vi "Electrical Measurements - Main.vi"() -> ()   [LabVIEW 2013]
doc: "Use this template to build a standard state machine design pattern. Each state executes code and determines which state to transition to. Contrast this design pattern with the User Interface Event Handler pattern, in which code executes in response to user actions. Contrast this design pattern also with the Queued Message Handler pattern, in which each message handling code can queue zero or more new messages."
uses:
  Controls/StateMachineStates 1.ctl
  Libraries/California Instruments iX Series/California Instruments iX Series.lvlib
  <instrlib>/California Instruments iX Series/Public/Data/Read Multiple Current Measurements.vi
panel:
  out "Waveform Graph":sgl[][](graph)
  out "Current Measurements 2":sgl[](array[numeric])
  out "Current Measurements":sgl[](array[numeric])
  out "multi-line string":string=":MEAS:CURR:AC?\n:MEAS:CURR:CRES?\n:MEAS:CURR:HARM:THD?\n:MEAS:POW:AC:REAL?\n:MEAS:POW:AC:APP?\n:MEAS:POW:AC:REAC?\n:MEAS:POW:AC:PFAC?\n:MEAS:POW:AC:TOT?\n:MEAS:VOLT:AC?\n:MEAS:VOLT:HARM:THD?"
  out "Waveforms":string[](array[string])
  out "Array":dbl[](array[numeric])
  in  "keep reading data/ stop and turn off":bool
  in  "Tab Control":T1(tab)
  in  "Enable Current Protection (Enabled)":bool
  in  "Current Level (0 A)":dbl=2.0
  in  "Current Protection Delay (0.1 Sec)":dbl=0.1
  in  "Voltage Mode (0: Fixed)":i32(ring) items=["Fixed", "Step", "Pulse", "List"]
  in  "Voltage Auto Level Control (0: On)":u16(ring) items=["On", "Off", "Regulation"]
  in  "Voltage Source (0:Internal)":u16(ring) items=["Internal", "External"]
  in  "Voltage Level (0V)":dbl=120.0
  in  "Transient Voltage Level (0V)":dbl
  in  "Voltage Protection Range (150V)":u16(ring)=150 items=["150"=150, "300"=300]
  in  "Voltage Limit (0.0 V)":dbl format="%.2g"
  in  "Phase (0°)":dbl
  in  "Triggered Phase (0°)":dbl
  in  "Phase Mode (0: Fixed)":i32(ring) items=["Fixed", "Step", "Pulse", "List"]
  in  "Frequency (60 Hz)":dbl=60.0
  in  "Triggered Frequency (60 Hz)":dbl=60.0
  in  "Frequency Mode (0: Fixed)":i32(ring) items=["Fixed", "Step", "Pulse", "List", "Sense", "External"]
  in  "Serial Configuration":cluster{"Baud Rate":u32, "Flow Control":u16}={"Baud Rate"=460800, "Flow Control"=0} {"Flow Control" items=["None", "XON/XOFF", "RTS/CTS", "XON/XOFF & RTS/CTS", "DTR/DSR", "XON/XOFF & DTR/DSR"]; "Baud Rate" items=["9600"=9600, "19200"=19200, "38400"=38400, "57600"=57600, "115200"=115200, "230400"=230400, "460800"=460800]}
  in  "VISA resource name":refnum<visa-resource-name>
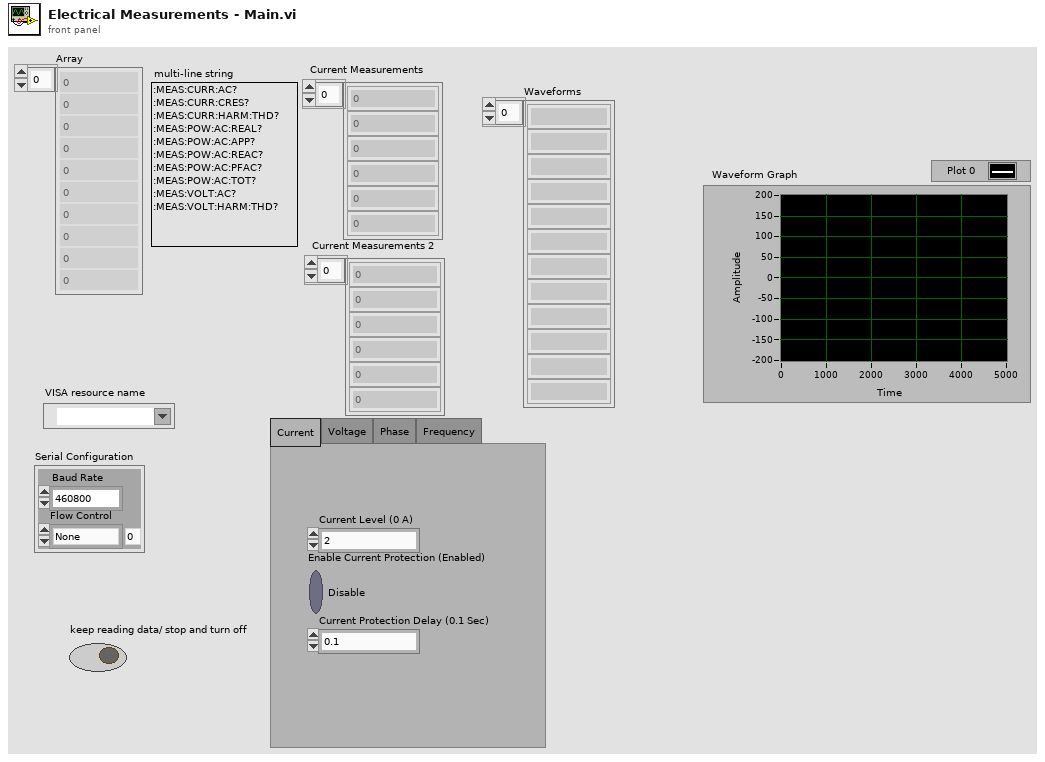
[diagram p1: front panel]
types:
  T1 = enum32{"Current", "Voltage", "Phase", "Frequency"}
  T2 = typedef "StateMachineStates 1.ctl" = enum16{"Idle", "Initialize", "turn supply on", "read electrical data", "read arb wave list", "read waveform data", "turn off light", "Stop"}
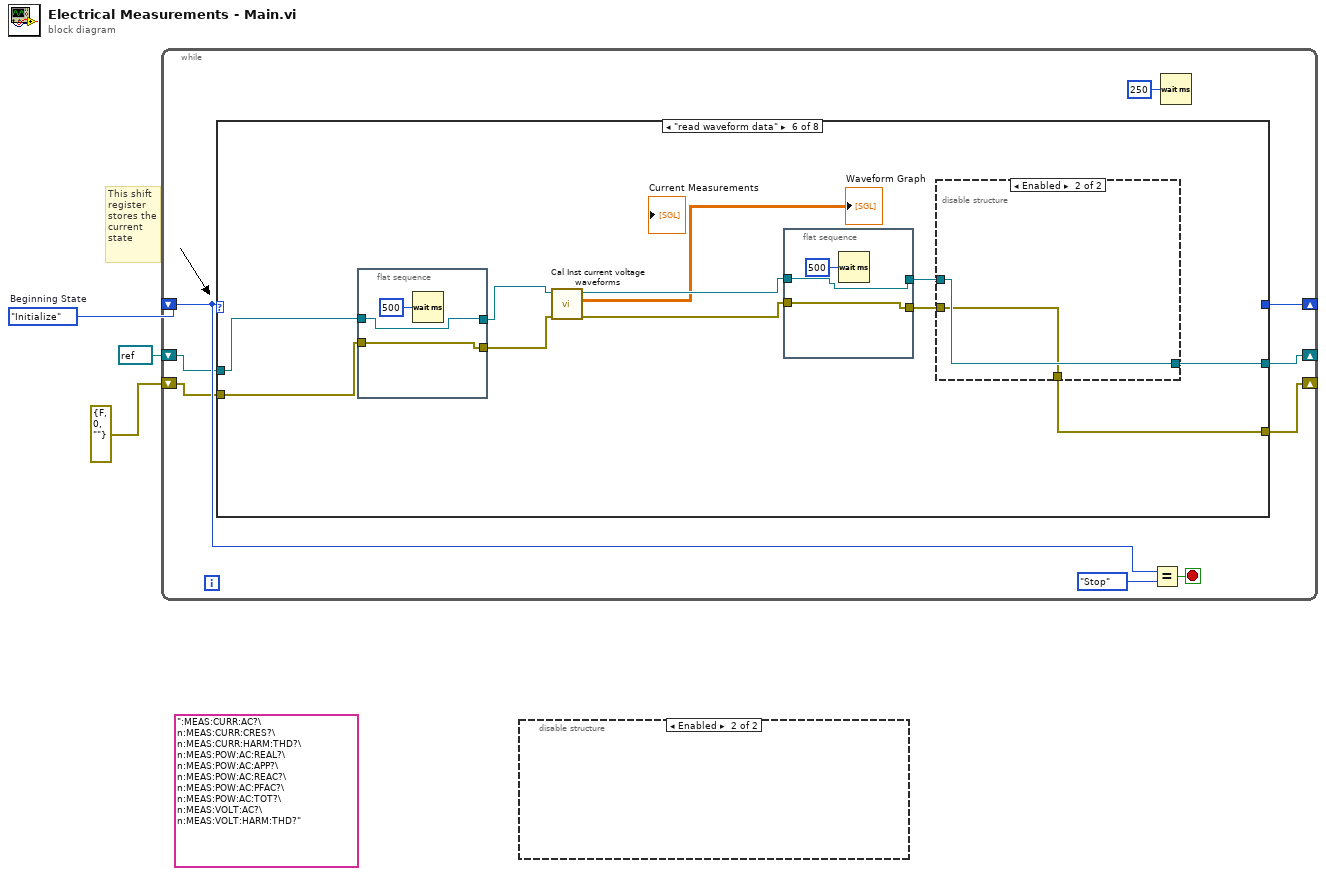
[diagram p0: block diagram]
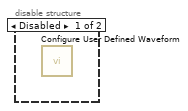
[diagram p2: hidden frame]
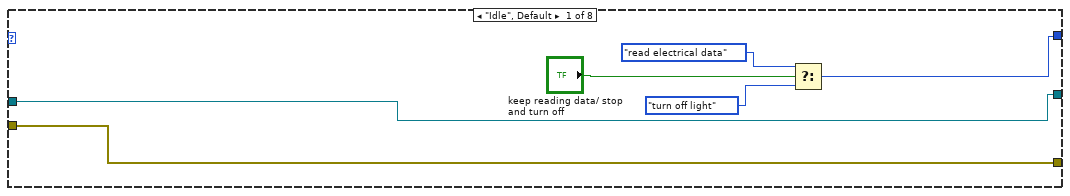
[diagram p3: hidden frame]
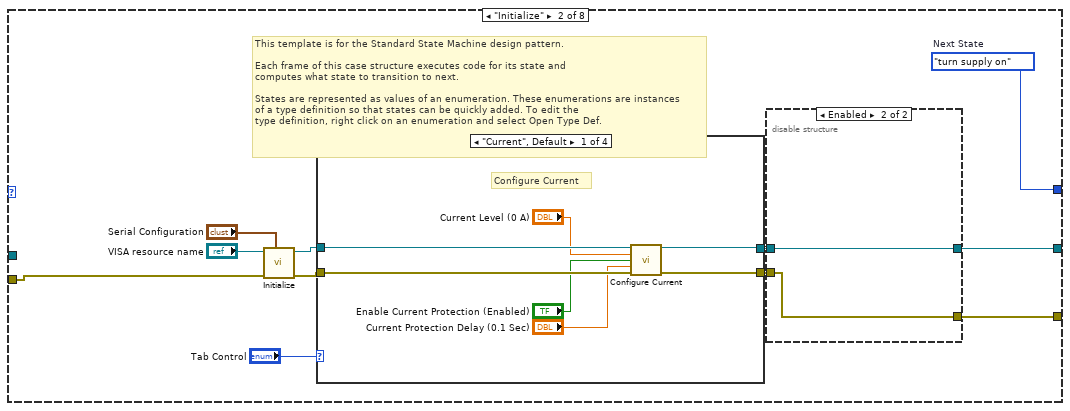
[diagram p4: hidden frame]
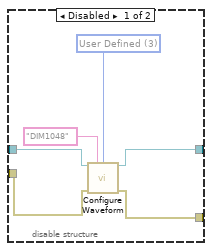
[diagram p5: hidden frame]
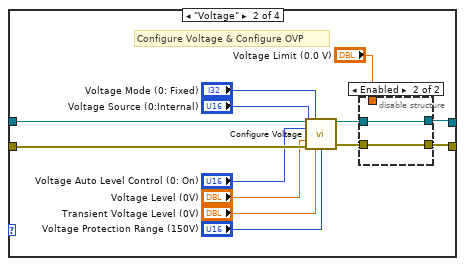
[diagram p6: hidden frame]
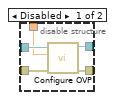
[diagram p7: hidden frame]
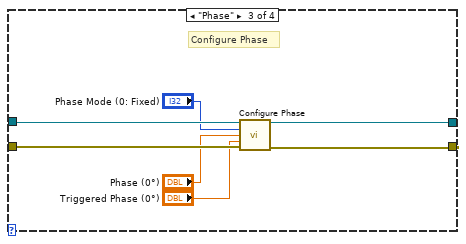
[diagram p8: hidden frame]
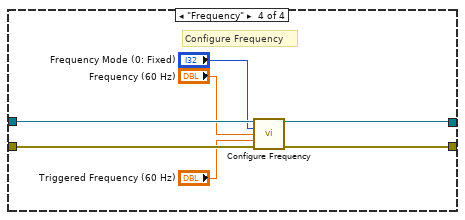
[diagram p9: hidden frame]
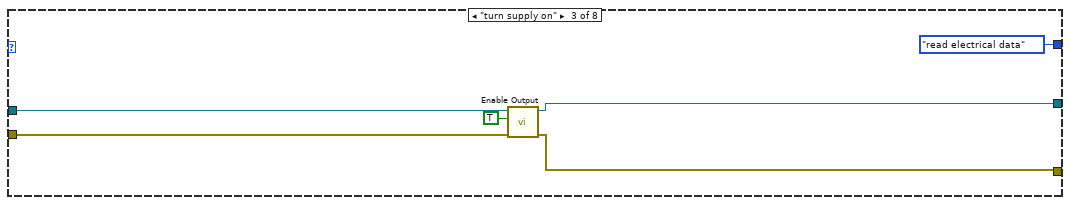
[diagram p10: hidden frame]
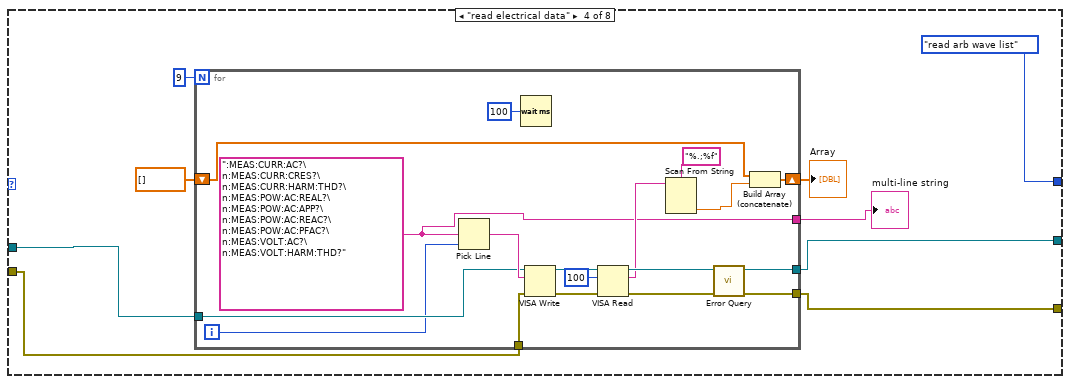
[diagram p11: hidden frame]
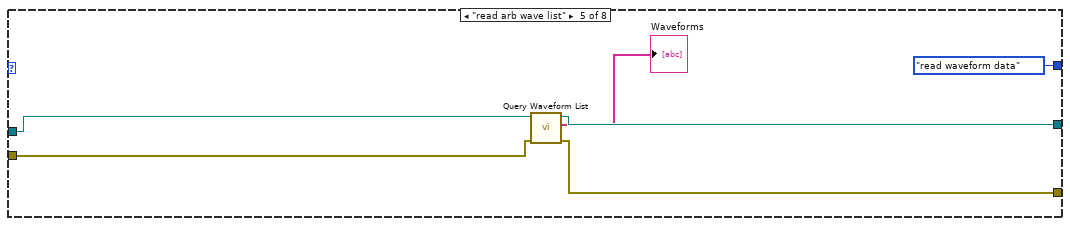
[diagram p12: hidden frame]
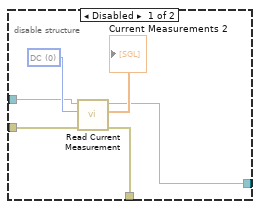
[diagram p13: hidden frame]
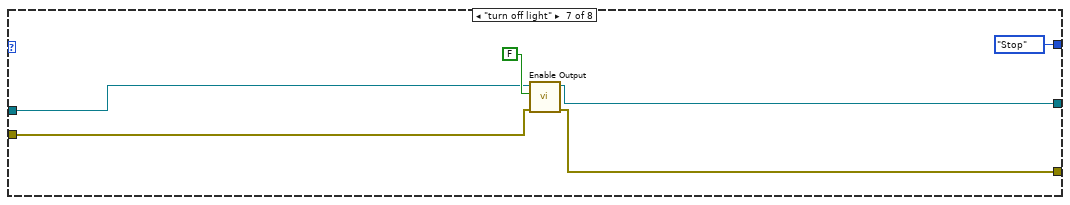
[diagram p14: hidden frame]
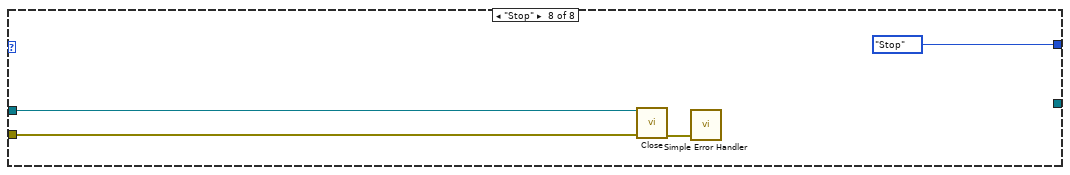
[diagram p15: hidden frame]
diagram:
  (unwired) ":MEAS:CURR:AC?\n:MEAS:CURR:CRES?\n:MEAS:CURR:HARM:THD?\n:MEAS:POW:AC:REAL?\n:MEAS:POW:AC:APP?\n:MEAS:POW:AC:REAC?\n:MEAS:POW:AC:PFAC?\n:MEAS:POW:AC:TOT?\n:MEAS:VOLT:AC?\n:MEAS:VOLT:HARM:THD?" ("multi-line string")
  w3 = StateMachineStates_1."Initialize"  # Beginning State
  # "This shift\nregister\nstores the\ncurrent\nstate"
  n1 = while {
    shift-right: [w9] -> _
    shift-left: w3 -> [w10]
    shift-right: [w5] -> _
    shift-left: refnum<visa-resource-name> refnum ("VISA resource name out") -> [w7]
    shift-right: [w4] -> _
    shift-left: errorcluster {"status"=FALSE, "code"=0, "source"=""} ("error out") -> [w6]
    stop <- w12 stop-if-true
    n2 = case shown="\"read waveform data\"" w10 {
      tunnel: [w15 w29 StateMachineStates_1."read electrical data" ("Next State") StateMachineStates_1."read arb wave list" ("Next State") StateMachineStates_1."read waveform data" ("Next State") _ StateMachineStates_1."Stop" ("Next State") StateMachineStates_1."Stop" ("Next State")] -> w9
      tunnel: w7 -> [w13 _ w84 w92 w117 w124 w145 w150]
      tunnel: w6 -> [w14 w23 w83 w91 w114 w123 w144 w149]
      tunnel: [w13 w20 w80 w89 w116 w126 w147 _] -> w5
      tunnel: [w14 w21 w79 w90 w115 w125 w146 _] -> w4
      frame "Idle", Default {
        n3 = Select(t=StateMachineStates_1."read electrical data" ("Next State"), s="keep reading data/ stop and turn off", f=StateMachineStates_1."turn off light" ("Next State")) -> (s? t:f=w15:T2)
      }
      frame "Initialize" {
        w29 = StateMachineStates_1."turn supply on"  # Next State
        # "This template is for the Standard State Machine design pattern.\n\nEach frame of this case structure executes code for its state and\ncomputes what state to transition to next.\n\nStates are represented as values of an enumeration. These enumerations are instances\nof a type definition so that states can be quickly added. To edit the \ntype definition, right click on an enumeration and select Open Type Def."
        n4 = call "Initialize.vi"("Serial Configuration"="Serial Configuration", "error in (no error)"=w23, "VISA resource name"="VISA resource name") -> ("error out"=w24:errorcluster, "VISA resource name out"=w25:refnum<visa-resource-name>)  [unwired: 7 in]
        n5 = case shown="\"Current\", Default" "Tab Control" {
          tunnel: w25 -> [w44 w57 w71 w78]
          tunnel: w24 -> [w43 w56 w70 w77]
          tunnel: [w39 w46 w66 w73] -> w19
          tunnel: [w38 w45 w65 w72] -> w22
          frame "Current", Default {
            # "Configure Current"
            n6 = call "Configure Current.vi"("VISA resource name"=w44, "Current Level (0 A)"="Current Level (0 A)", "Enable Current Protection (Enabled)"="Enable Current Protection (Enabled)", "Current Protection Delay (0.1 Sec)"="Current Protection Delay (0.1 Sec)", "error in (no error)"=w43) -> ("VISA resource name out"=w39:refnum<visa-resource-name>, "error out"=w38:errorcluster)  [unwired: 9 in]
          }
          frame "Voltage" {
            # "Configure Voltage & Configure OVP"
            n7 = call "Configure Voltage.vi"("VISA resource name"=w57, "Voltage Mode (0: Fixed)"="Voltage Mode (0: Fixed)", "Voltage Auto Level Control (0: On)"="Voltage Auto Level Control (0: On)", "Voltage Source (0:Internal)"="Voltage Source (0:Internal)", "Voltage Level (0V)"="Voltage Level (0V)", "error in (no error)"=w56, "Transient Voltage Level (0V)"="Transient Voltage Level (0V)", "Voltage Protection Range (150V)"="Voltage Protection Range (150V)") -> ("VISA resource name out"=w49:refnum<visa-resource-name>, "error out"=w48:errorcluster)  [unwired: 6 in]
            n8 = disable-structure shown="Enabled" {
              disable-tunnel: w49 -> [w62 w64]
              disable-tunnel: w48 -> [w61 w63]
              disable-tunnel: "Voltage Limit (0.0 V)" -> [w60 _]
              disable-tunnel: [w59 w64] -> w46
              disable-tunnel: [w58 w63] -> w45
              frame Disabled {
                n9 = call "Configure OVP.vi"("error in (no error)"=w61, "Voltage Limit (0.0 V)"=w60, "VISA resource name"=w62) -> ("error out"=w58:errorcluster, "VISA resource name out"=w59:refnum<visa-resource-name>)  [unwired: 7 in]
              }
              frame Enabled {
              }
            }
          }
          frame "Phase" {
            # "Configure Phase"
            n10 = call "Configure Phase.vi"("VISA resource name"=w71, "Phase Mode (0: Fixed)"="Phase Mode (0: Fixed)", "Phase (0°)"="Phase (0°)", "Triggered Phase (0°)"="Triggered Phase (0°)", "error in (no error)"=w70) -> ("VISA resource name out"=w66:refnum<visa-resource-name>, "error out"=w65:errorcluster)  [unwired: 9 in]
          }
          frame "Frequency" {
            # "Configure Frequency"
            n11 = call "Configure Frequency.vi"("VISA resource name"=w78, "Frequency Mode (0: Fixed)"="Frequency Mode (0: Fixed)", "Frequency (60 Hz)"="Frequency (60 Hz)", "Triggered Frequency (60 Hz)"="Triggered Frequency (60 Hz)", "error in (no error)"=w77) -> ("VISA resource name out"=w73:refnum<visa-resource-name>, "error out"=w72:errorcluster)  [unwired: 9 in]
          }
        }
        n12 = disable-structure shown="Enabled" {
          disable-tunnel: w22 -> [w35 w36]
          disable-tunnel: [w34 w36] -> w21
          disable-tunnel: [w33 w37] -> w20
          disable-tunnel: w19 -> [w32 w37]
          frame Disabled {
            w31 = u16 3 items=["Sinusoid", "Square", "Clipped Sinusiod", "User Defined"] ("Waveform Type (0:Sinusoid)")
            n13 = call <instrlib>:"Configure Waveform.vi"("VISA resource name"=w32, "Waveform Name (\"ARB1\")"="DIM1048" ("Waveform Name (\"ARB1\")"), "Waveform Type (0:Sinusoid)"=w31, "error in (no error)"=w35) -> ("VISA resource name out"=w33:refnum<visa-resource-name>, "error out"=w34:errorcluster)  [unwired: 10 in]
          }
          frame Enabled {
          }
        }
      }
      frame "turn supply on" {
        n14 = call "Enable Output.vi"("error in (no error)"=w83, "Enable Output (T: Enable)"=TRUE, "VISA resource name"=w84) -> ("error out"=w79:errorcluster, "VISA resource name out"=w80:refnum<visa-resource-name>)  [unwired: 7 in]
      }
      frame "read electrical data" {
        n15 = for {
          N: 9 -> [_]
          tunnel: [w111] -> w90
          tunnel: [w110] -> w89
          tunnel: w92 -> [w101]
          tunnel: w91 -> [w100]
          shift-right: [w99] -> w87
          shift-left: dbl[] [] -> [w98]
          tunnel: [w95] -> w85
          i -> [w96]
          w95 = ":MEAS:CURR:AC?\n:MEAS:CURR:CRES?\n:MEAS:CURR:HARM:THD?\n:MEAS:POW:AC:REAL?\n:MEAS:POW:AC:APP?\n:MEAS:POW:AC:REAC?\n:MEAS:POW:AC:PFAC?\n:MEAS:VOLT:AC?\n:MEAS:VOLT:HARM:THD?" ("multi-line string")
          n16 = Pick Line(multi-line string=w95, line index=w96) -> (output string=w102:string)  [unwired: 1 in]
          n17 = Wait (ms)(milliseconds to wait=u32 100) -> ()  [unwired: 1 out]
          n18 = VISA Write(VISA resource name=w101, write buffer=w102, error in (no error)=w100) -> (VISA resource name out=w109:refnum<visa-resource-name>, error out=w108:errorcluster)  [unwired: 1 out]
          n19 = VISA Read(VISA resource name=w109, byte count=u32 100, error in (no error)=w108) -> (VISA resource name out=w107:refnum<visa-resource-name>, read buffer=w104:string, error out=w106:errorcluster)  [unwired: 1 out]
          n20 = Scan From String(format string="%.;%f", input string=w104) -> (output 1=w97:dbl)  [unwired: 3 in, 3 out]
          n21 = call "Error Query.vi"("error in (no error)"=w106, "VISA resource name"=w107) -> ("error out"=w111:errorcluster, "VISA resource name out"=w110:refnum<visa-resource-name>)  [unwired: 6 in, 2 out]
          n22 = Build Array (concatenate)(w98, w97) -> (w99:dbl[])
        }
        "Array" <- w87
        "multi-line string" <- w85
      }
      frame "read arb wave list" {
        n23 = call "Query Waveform List.vi"("error in (no error)"=w114, "VISA resource name"=w117) -> ("error out"=w115:errorcluster, "Waveforms"=→"Waveforms":string[], "VISA resource name out"=w116:refnum<visa-resource-name>)  [unwired: 7 in]
      }
      frame "read waveform data" {
        n24 = flat-sequence {
          tunnel: w124 -> [w130]
          tunnel: [w130] -> w122
          tunnel: [w129] -> w121
          tunnel: w123 -> [w129]
          frame #0 {
            n25 = Wait (ms)(milliseconds to wait=u32 500) -> ()  [unwired: 1 out]
          }
        }
        n26 = call "Cal Inst current voltage waveforms.vi"("error in (no error)"=w121, "VISA resource name"=w122) -> ("error out"=w120:errorcluster, "Waveform Graph"=→"Waveform Graph":sgl[][], "VISA resource name out"=w119:refnum<visa-resource-name>)  [unwired: 7 in]
        n27 = flat-sequence {
          tunnel: w119 -> [w141]
          tunnel: [w141] -> w128
          tunnel: [w140] -> w127
          tunnel: w120 -> [w140]
          frame #0 {
            n28 = Wait (ms)(milliseconds to wait=u32 500) -> ()  [unwired: 1 out]
          }
        }
        n29 = disable-structure shown="Enabled" {
          disable-tunnel: w128 -> [w135 w139]
          disable-tunnel: w127 -> [w134 w138]
          disable-tunnel: [w133 w139] -> w126
          disable-tunnel: [w132 w138] -> w125
          frame Disabled {
            w137 = u16 0 items=["DC", "Current Harmonic Amplitude", "Current Harmonic Phase", "Neutral DC Current", "Neutral Current Harmonic Amplitude", "Neutral Current Harmonic Phase"] ("Multiple Current Measurement Type (0:DC)")
            n30 = call-poly <instrlib>:"Read Current Measurement.vi"("error in (no error)"=w134, "Multiple Current Measurement Type (0:DC)"=w137, "VISA resource name"=w135) -> ("error out"=w132:errorcluster, "Current Measurements"=→"Current Measurements 2":sgl[], "VISA resource name out"=w133:refnum<visa-resource-name>)  [unwired: 6 in]
          }
          frame Enabled {
          }
        }
      }
      frame "turn off light" {
        n31 = call "Enable Output.vi"("error in (no error)"=w144, "Enable Output (T: Enable)"=FALSE, "VISA resource name"=w145) -> ("error out"=w146:errorcluster, "VISA resource name out"=w147:refnum<visa-resource-name>)  [unwired: 7 in]
      }
      frame "Stop" {
        n32 = call "Close.vi"("error in (no error)"=w149, "VISA resource name"=w150) -> ("error out"=w151:errorcluster)  [unwired: 9 in]
        n33 = call <vilib>:"Simple Error Handler.vi"("error in (no error)"=w151) -> ()  [unwired: 4 in, 5 out]
      }
    }
    n34 = Equal?(x=w10, y=StateMachineStates_1."Stop" ("States")) -> (x = y?=w12:bool)
    n35 = Wait (ms)(milliseconds to wait=u32 250) -> ()  [unwired: 1 out]
  }
  n36 = disable-structure shown="Enabled" {
    frame Disabled {
      n37 = call <instrlib>:"Configure User Defined Waveform.vi"() -> ()  [unwired: 14 in, 2 out]
    }
    frame Enabled {
    }
  }
